vi "rsscope_core_global.vi"() -> ()   [LabVIEW 2018] (continued)
"Write Callback"="", "Supported Models"="", "Instrument Options"="K4", "Flags"=0, "Help"="Specifies a step to trigger on each n-th cycle inside the given range. This allows for specific triggering if slot multiplexing is used.\n\nAvailable Repeated Capabilities:\nTrigger: TrigA, TrigB, TrigR\r\n\nRemote-control command(s):\nTRIGger<m>:FLXRay:CSTep"}, {"Level"=3, "Class Only"=FALSE, "Identifier"="RSSCOPE_ATTR_PROTOCOL_FLEXRAY_TRIGGER_SYMBOL", "Descriptive Name"="Protocol FlexRay Trigger Symbol", "Data Type"=0, "Command"="TRIG{Trigger}:FLXR:SYMB", "Access"=2, "Range Table"="rsscope_rngFlexRaySymbol", "Read Callback"="", "Write Callback"="", "Supported Models"="", "Instrument Options"="K4", "Flags"=0, "Help"="Selects the trigger on symbol or on a wakeup pattern.\n\nAvailable Repeated Capabilities:\nTrigger: TrigA, TrigB, TrigR\r\n\nRemote-control command(s):\nTRIGger<m>:FLXRay:SYMBol"}, {"Level"=3, "Class Only"=TRUE, "Identifier"="", "Descriptive Name"="Indicator Bits", "Data Type"=0, "Command"="", "Access"=0, "Range Table"="", "Read Callback"="", "Write Callback"="", "Supported Models"="", "Instrument Options"="", "Flags"=0, "Help"="Configures indicator bits."}, {"Level"=4, "Class Only"=FALSE, "Identifier"="RSSCOPE_ATTR_PROTOCOL_FLEXRAY_TRIGGER_PAYLOAD_PREAMBLE", "Descriptive Name"="Protocol FlexRay Trigger Payload Preamble", "Data Type"=0, "Command"="TRIG{Trigger}:FLXR:PLPR", "Access"=2, "Range Table"="rsscope_rngFlexRayIndicatorBits", "Read Callback"="", "Write Callback"="", "Supported Models"="", "Instrument Options"="K4", "Flags"=0, "Help"="Triggers on the payload preamble indicator bit that indicates a Network Management Vector in the payload segment.\n\nAvailable Repeated Capabilities:\nTrigger: TrigA, TrigB, TrigR\r\n\nRemote-control command(s):\nTRIGger<m>:FLXRay:PLPReamble"}, {"Level"=4, "Class Only"=FALSE, "Identifier"="RSSCOPE_ATTR_PROTOCOL_FLEXRAY_TRIGGER_NULL_FRAME", "Descriptive Name"="Protocol FlexRay Trigger Null Frame", "Data Type"=0, "Command"="TRIG{Trigger}:FLXR:NUFR", "Access"=2, "Range Table"="rsscope_rngFlexRayIndicatorBits", "Read Callback"="", "Write Callback"="", "Supported Models"="", "Instrument Options"="K4", "Flags"=0, "Help"="Triggers on the null frame indicator bit, a frame without usable data.\n\nAvailable Repeated Capabilities:\nTrigger: TrigA, TrigB, TrigR\r\n\nRemote-control command(s):\nTRIGger<m>:FLXRay:NUFRame"}, {"Level"=4, "Class Only"=FALSE, "Identifier"="RSSCOPE_ATTR_PROTOCOL_FLEXRAY_TRIGGER_SYNC_FRAME", "Descriptive Name"="Protocol FlexRay Trigger Sync Frame", "Data Type"=0, "Command"="TRIG{Trigger}:FLXR:SYFR", "Access"=2, "Range Table"="rsscope_rngFlexRayIndicatorBits", "Read Callback"="", "Write Callback"="", "Supported Models"="", "Instrument Options"="K4", "Flags"=0, "Help"="Triggers on the sync frame used for synchronization of the FlexRay system. Only sync nodes can send this frame type.\n\nAvailable Repeated Capabilities:\nTrigger: TrigA, TrigB, TrigR\r\n\nRemote-control command(s):\nTRIGger<m>:FLXRay:SYFRame"}, {"Level"=4, "Class Only"=FALSE, "Identifier"="RSSCOPE_ATTR_PROTOCOL_FLEXRAY_TRIGGER_STARTUP_FRAME", "Descriptive Name"="Protocol FlexRay Trigger Startup Frame", "Data Type"=0, "Command"="TRIG{Trigger}:FLXR:STFR", "Access"=2, "Range Table"="rsscope_rngFlexRayIndicatorBits", "Read Callback"="", "Write Callback"="", "Supported Models"="", "Instrument Options"="K4", "Flags"=0, "Help"="Triggers on startup frames used for startup of the network. Only specific start nodes can send this frame type.\n\nAvailable Repeated Capabilities:\nTrigger: TrigA, TrigB, TrigR\r\n\nRemote-control command(s):\nTRIGger<m>:FLXRay:STFRame"}, {"Level"=3, "Class Only"=TRUE, "Identifier"="", "Descriptive Name"="Frame", "Data Type"=0, "Command"="", "Access"=0, "Range Table"="", "Read Callback"="", "Write Callback"="", "Supported Models"="", "Instrument Options"="", "Flags"=0, "Help"="Configures Flex Ray frame."}, {"Level"=4, "Class Only"=FALSE, "Identifier"="RSSCOPE_ATTR_PROTOCOL_FLEXRAY_TRIGGER_FRAME_CONDITION", "Descriptive Name"="Protocol FlexRay Trigger Frame Condition", "Data Type"=0, "Command"="TRIG{Trigger}:FLXR:FCON", "Access"=2, "Range Table"="rsscope_rngFlexRayCondition", "Read Callback"="", "Write Callback"="", "Supported Models"="", "Instrument Options"="K4", "Flags"=0, "Help"="Sets the operator to set a frame ID or a frame ID range.\n\nAvailable Repeated Capabilities:\nTrigger: TrigA, TrigB, TrigR\r\n\nRemote-control command(s):\nTRIGger<m>:FLXRay:FCONdition"}, {"Level"=4, "Class Only"=FALSE, "Identifier"="RSSCOPE_ATTR_PROTOCOL_FLEXRAY_TRIGGER_PATTERN_FRAME_MIN", "Descriptive Name"="Protocol FlexRay Trigger Pattern Frame Min", "Data Type"=2, "Command"="TRIG{Trigger}:FLXR:FMIN", "Access"=2, "Range Table"="", "Read Callback"="", "Write Callback"="", "Supported Models"="", "Instrument Options"="K4", "Flags"=0, "Help"="Specifies a frame identifier pattern - the number of the slot - or sets the start value of an identifier range.\n\nAvailable Repeated Capabilities:\nTrigger: TrigA, TrigB, TrigR\r\n\nRemote-control command(s):\nTRIGger<m>:FLXRay:FMIN"}, {"Level"=4, "Class Only"=FALSE, "Identifier"="RSSCOPE_ATTR_PROTOCOL_FLEXRAY_TRIGGER_PATTERN_FRAME_MAX", "Descriptive Name"="Protocol FlexRay Trigger Pattern Frame Max", "Data Type"=2, "Command"="TRIG{Trigger}:FLXR:FMAX", "Access"=2, "Range Table"="", "Read Callback"="", "Write Callback"="", "Supported Models"="", "Instrument Options"="K4", "Flags"=0, "Help"="Sets the end value of an identifier range.\n\nAvailable Repeated Capabilities:\nTrigger: TrigA, TrigB, TrigR\r\n\nRemote-control command(s):\nTRIGger<m>:FLXRay:FMAX"}, {"Level"=3, "Class Only"=TRUE, "Identifier"="", "Descriptive Name"="Data", "Data Type"=0, "Command"="", "Access"=0, "Range Table"="", "Read Callback"="", "Write Callback"="", "Supported Models"="", "Instrument Options"="", "Flags"=0, "Help"="Configures Flex ray data."}, {"Level"=4, "Class Only"=FALSE, "Identifier"="RSSCOPE_ATTR_PROTOCOL_FLEXRAY_TRIGGER_DATA_CONDITION", "Descriptive Name"="Protocol FlexRay Trigger Data Condition", "Data Type"=0, "Command"="TRIG{Trigger}:FLXR:DCON", "Access"=2, "Range Table"="rsscope_rngFlexRayCondition", "Read Callback"="", "Write Callback"="", "Supported Models"="", "Instrument Options"="K4", "Flags"=0, "Help"="Sets the operator to set a specific data pattern or a data pattern range.\n\nAvailable Repeated Capabilities:\nTrigger: TrigA, TrigB, TrigR\r\n\nRemote-control command(s):\nTRIGger<m>:FLXRay:DCONdition"}, {"Level"=4, "Class Only"=FALSE, "Identifier"="RSSCOPE_ATTR_PROTOCOL_FLEXRAY_TRIGGER_PATTERN_DATA_MIN", "Descriptive Name"="Protocol FlexRay Trigger Pattern Data Min", "Data Type"=2, "Command"="TRIG{Trigger}:FLXR:DMIN", "Access"=2, "Range Table"="", "Read Callback"="", "Write Callback"="", "Supported Models"="", "Instrument Options"="K4", "Flags"=0, "Help"="Specifies a data pattern, or sets the start value of a data pattern range.\n\nAvailable Repeated Capabilities:\nTrigger: TrigA, TrigB, TrigR\r\n\nRemote-control command(s):\nTRIGger<m>:FLXRay:DMIN"}, {"Level"=4, "Class Only"=FALSE, "Identifier"="RSSCOPE_ATTR_PROTOCOL_FLEXRAY_TRIGGER_PATTERN_DATA_MAX", "Descriptive Name"="Protocol FlexRay Trigger Pattern Data Max", "Data Type"=2, "Command"="TRIG{Trigger}:FLXR:DMAX", "Access"=2, "Range Table"="", "Read Callback"="", "Write Callback"="", "Supported Models"="", "Instrument Options"="K4", "Flags"=0, "Help"="Sets the end value of an data range.\n\nAvailable Repeated Capabilities:\nTrigger: TrigA, TrigB, TrigR\r\n\nRemote-control command(s):\nTRIGger<m>:FLXRay:DMAX"}, {"Level"=3, "Class Only"=TRUE, "Identifier"="", "Descriptive Name"="Payload Length", "Data Type"=0, "Command"="", "Access"=0, "Range Table"="", "Read Callback"="", "Write Callback"="", "Supported Models"="", "Instrument Options"="", "Flags"=0, "Help"="Configures Flex Ray Payload Length."}, {"Level"=4, "Class Only"=FALSE, "Identifier"="RSSCOPE_ATTR_PROTOCOL_FLEXRAY_TRIGGER_PAYLOAD_LENGTH_CONDITION", "Descriptive Name"="Protocol FlexRay Trigger Payload Length Condition", "Data Type"=0, "Command"="TRIG{Trigger}:FLXR:PCON", "Access"=2, "Range Table"="rsscope_rngFlexRayCondition", "Read Callback"="", "Write Callback"="", "Supported Models"="", "Instrument Options"="K4", "Flags"=0, "Help"="Sets the operator for the payload length trigger setting. You can defined an exact value, or a range.\n\nAvailable Repeated Capabilities:\nTrigger: TrigA, TrigB, TrigR\r\n\nRemote-control command(s):\nTRIGger<m>:FLXRay:PCONdition"}, {"Level"=4, "Class Only"=FALSE, "Identifier"="RSSCOPE_ATTR_PROTOCOL_FLEXRAY_TRIGGER_PAYLOAD_MIN", "Descriptive Name"="Protocol FlexRay Trigger Payload Min", "Data Type"=0, "Command"="TRIG{Trigger}:FLXR:PMIN", "Access"=2, "Range Table"="rsscope_rngFlexRayPayloadMinMax", "Read Callback"="", "Write Callback"="", "Supported Models"="", "Instrument Options"="K4", "Flags"=0, "Help"="Specifies a payload length - the number of words in the payload segment - or sets the start value of an payload length range. Information is transmitted in 2-byte words, so the number of data bytes in the payload segment is twice the payload length.\n\nAvailable Repeated Capabilities:\nTrigger: TrigA, TrigB, TrigR\r\n\nRemote-control command(s):\nTRIGger<m>:FLXRay:PMIN"}, {"Level"=4, "Class Only"=FALSE, "Identifier"="RSSCOPE_ATTR_PROTOCOL_FLEXRAY_TRIGGER_PAYLOAD_MAX", "Descriptive Name"="Protocol FlexRay Trigger Payload Max", "Data Type"=0, "Command"="TRIG{Trigger}:FLXR:PMAX", "Access"=2, "Range Table"="rsscope_rngFlexRayPayloadMinMax", "Read Callback"="", "Write Callback"="", "Supported Models"="", "Instrument Options"="K4", "Flags"=0, "Help"="Sets the end value of a payload length range.\n\nAvailable Repeated Capabilities:\nTrigger: TrigA, TrigB, TrigR\r\n\nRemote-control command(s):\nTRIGger<m>:FLXRay:PMAX"}, {"Level"=3, "Class Only"=TRUE, "Identifier"="", "Descriptive Name"="Cycle Count", "Data Type"=0, "Command"="", "Access"=0, "Range Table"="", "Read Callback"="", "Write Callback"="", "Supported Models"="", "Instrument Options"="", "Flags"=0, "Help"="Configures Flex Ray Cycle Count."}, {"Level"=4, "Class Only"=FALSE, "Identifier"="RSSCOPE_ATTR_PROTOCOL_FLEXRAY_TRIGGER_CYCLE_COUNT_CONDITION", "Descriptive Name"="Protocol FlexRay Trigger Cycle Count Condition", "Data Type"=0, "Command"="TRIG{Trigger}:FLXR:CEN", "Access"=2, "Range Table"="rsscope_rngFlexRayCondition", "Read Callback"="", "Write Callback"="", "Supported Models"="", "Instrument Options"="K4", "Flags"=0, "Help"="Sets the operator to define a cycle count or a cycle count range.\n\nAvailable Repeated Capabilities:\nTrigger: TrigA, TrigB, TrigR\r\n\nRemote-control command(s):\nTRIGger<m>:FLXRay:CENable"}, {"Level"=4, "Class Only"=FALSE, "Identifier"="RSSCOPE_ATTR_PROTOCOL_FLEXRAY_TRIGGER_CYCLE_MIN", "Descriptive Name"="Protocol FlexRay Trigger Cycle Min", "Data Type"=0, "Command"="TRIG{Trigger}:FLXR:CMIN", "Access"=2, "Range Table"="rsscope_rngFlexRayCycleMinMax", "Read Callback"="", "Write Callback"="", "Supported Models"="", "Instrument Options"="K4", "Flags"=0, "Help"="Specifies a cycle count - the number of the current FlexRay cycle - or sets the start value of an cycle count range.\n\nAvailable Repeated Capabilities:\nTrigger: TrigA, TrigB, TrigR\r\n\nRemote-control command(s):\nTRIGger<m>:FLXRay:CMIN"}, {"Level"=4, "Class Only"=FALSE, "Identifier"="RSSCOPE_ATTR_PROTOCOL_FLEXRAY_TRIGGER_CYCLE_MAX", "Descriptive Name"="Protocol FlexRay Trigger Cycle Max", "Data Type"=0, "Command"="TRIG{Trigger}:FLXR:CMAX", "Access"=2, "Range Table"="rsscope_rngFlexRayCycleMinMax", "Read Callback"="", "Write Callback"="", "Supported Models"="", "Instrument Options"="K4", "Flags"=0, "Help"="Sets the end value of a cycle count range.\n\nAvailable Repeated Capabilities:\nTrigger: TrigA, TrigB, TrigR\r\n\nRemote-control command(s):\nTRIGger<m>:FLXRay:CMAX"}, {"Level"=3, "Class Only"=TRUE, "Identifier"="", "Descriptive Name"="Data Position", "Data Type"=0, "Command"="", "Access"=0, "Range Table"="", "Read Callback"="", "Write Callback"="", "Supported Models"="", "Instrument Options"="", "Flags"=0, "Help"="Configures Flex Ray Data Position."}, {"Level"=4, "Class Only"=FALSE, "Identifier"="RSSCOPE_ATTR_PROTOCOL_FLEXRAY_TRIGGER_DATA_POSITION_CONDITION", "Descriptive Name"="Protocol FlexRay Trigger Data Position Condition", "Data Type"=0, "Command"="TRIG{Trigger}:FLXR:DPOP", "Access"=2, "Range Table"="rsscope_rngFlexRayCondition", "Read Callback"="", "Write Callback"="", "Supported Models"="", "Instrument Options"="K4", "Flags"=0, "Help"="Sets the operator for the data position. You can defined an exact position, or a position range.\n\nAvailable Repeated Capabilities:\nTrigger: TrigA, TrigB, TrigR\r\n\nRemote-control command(s):\nTRIGger<m>:FLXRay:DPOPerator"}, {"Level"=4, "Class Only"=FALSE, "Identifier"="RSSCOPE_ATTR_PROTOCOL_FLEXRAY_TRIGGER_DATA_POSITION_MIN", "Descriptive Name"="Protocol FlexRay Trigger Data Position Min", "Data Type"=0, "Command"="TRIG{Trigger}:FLXR:DPOS", "Access"=2, "Range Table"="rsscope_rngFlexRayPositionMinMax", "Read Callback"="", "Write Callback"="", "Supported Models"="", "Instrument Options"="K4", "Flags"=0, "Help"="Sets the number of data bytes to be skipped after start of the payload segment.\n\nAvailable Repeated Capabilities:\nTrigger: TrigA, TrigB, TrigR\r\n\nRemote-control command(s):\nTRIGger<m>:FLXRay:DPOSition"}, {"Level"=4, "Class Only"=FALSE, "Identifier"="RSSCOPE_ATTR_PROTOCOL_FLEXRAY_TRIGGER_DATA_POSITION_MAX", "Descriptive Name"="Protocol FlexRay Trigger Data Position Max", "Data Type"=0, "Command"="TRIG{Trigger}:FLXR:DPTO", "Access"=2, "Range Table"="rsscope_rngFlexRayPositionMinMax", "Read Callback"="", "Write Callback"="", "Supported Models"="", "Instrument Options"="K4", "Flags"=0, "Help"="Defines the last byte of interest.\n\nAvailable Repeated Capabilities:\nTrigger: TrigA, TrigB, TrigR\r\n\nRemote-control command(s):\nTRIGger<m>:FLXRay:DPTO"}, {"Level"=3, "Class Only"=TRUE, "Identifier"="", "Descriptive Name"="Error Conditions", "Data Type"=0, "Command"="", "Access"=0, "Range Table"="", "Read Callback"="", "Write Callback"="", "Supported Models"="", "Instrument Options"="", "Flags"=0, "Help"="Triggers on one or more errors in the frame."}, {"Level"=4, "Class Only"=FALSE, "Identifier"="RSSCOPE_ATTR_PROTOCOL_FLEXRAY_TRIGGER_FRAME_START_SEQUENCE_ERROR", "Descriptive Name"="Protocol FlexRay Trigger Frame Start Sequence Error", "Data Type"=3, "Command"="TRIG{Trigger}:FLXR:FSS", "Access"=2, "Range Table"="", "Read Callback"="", "Write Callback"="", "Supported Models"="", "Instrument Options"="K4", "Flags"=0, "Help"="Triggers on Error in a Frame Start Sequence. FSS follows the Transmission Start Sequence TSS at the beginning of each frame.\n\nAvailable Repeated Capabilities:\nTrigger: TrigA, TrigB, TrigR\r\n\nRemote-control command(s):\nTRIGger<m>:FLXRay:FSSerror"}, {"Level"=4, "Class Only"=FALSE, "Identifier"="RSSCOPE_ATTR_PROTOCOL_FLEXRAY_TRIGGER_BYTE_START_SEQUENCE_ERROR", "Descriptive Name"="Protocol FlexRay Trigger Byte Start Sequence Error", "Data Type"=3, "Command"="TRIG{Trigger}:FLXR:BSS", "Access"=2, "Range Table"="", "Read Callback"="", "Write Callback"="", "Supported Models"="", "Instrument Options"="K4", "Flags"=0, "Help"="Triggers on error in SyteStart Sequence. The BSS is transmitted before each byte.\n\nAvailable Repeated Capabilities:\nTrigger: TrigA, TrigB, TrigR\r\n\nRemote-control command(s):\nTRIGger<m>:FLXRay:BSSerror"}, {"Level"=4, "Class Only"=FALSE, "Identifier"="RSSCOPE_ATTR_PROTOCOL_FLEXRAY_TRIGGER_FRAME_END_SEQUENCE_ERROR", "Descriptive Name"="Protocol FlexRay Trigger Frame End Sequence Error", "Data Type"=3, "Command"="TRIG{Trigger}:FLXR:FES", "Access"=2, "Range Table"="", "Read Callback"="", "Write Callback"="", "Supported Models"="", "Instrument Options"="K4", "Flags"=0, "Help"="Triggers on error in Frame End Sequence. FES indicates the end of each frame.\n\nAvailable Repeated Capabilities:\nTrigger: TrigA, TrigB, TrigR\r\n\nRemote-control command(s):\nTRIGger<m>:FLXRay:FESerror"}, {"Level"=4, "Class Only"=FALSE, "Identifier"="RSSCOPE_ATTR_PROTOCOL_FLEXRAY_TRIGGER_HEADER_CRC_ERROR", "Descriptive Name"="Protocol FlexRay Trigger Header CRC Error", "Data Type"=3, "Command"="TRIG{Trigger}:FLXR:HCRC", "Access"=2, "Range Table"="", "Read Callback"="", "Write Callback"="", "Supported Models"="", "Instrument Options"="K4", "Flags"=0, "Help"="Triggers on error in the Cyclic Redundancy Check of the header data (mainly frame ID and payload length).\n\nAvailable Repeated Capabilities:\nTrigger: TrigA, TrigB, TrigR\r\n\nRemote-control command(s):\nTRIGger<m>:FLXRay:HCRCerror"}, {"Level"=4, "Class Only"=FALSE, "Identifier"="RSSCOPE_ATTR_PROTOCOL_FLEXRAY_TRIGGER_PAYLOAD_CRC_ERROR", "Descriptive Name"="Protocol FlexRay Trigger Payload CRC Error", "Data Type"=3, "Command"="TRIG{Trigger}:FLXR:PCRC", "Access"=2, "Range Table"="", "Read Callback"="", "Write Callback"="", "Supported Models"="", "Instrument Options"="K4", "Flags"=0, "Help"="Triggers on error in the Cyclic Redundancy Check of the payload data.\n\nAvailable Repeated Capabilities:\nTrigger: TrigA, TrigB, TrigR\r\n\nRemote-control command(s):\nTRIGger<m>:FLXRay:PCRCerror"}, {"Level"=2, "Class Only"=TRUE, "Identifier"="", "Descriptive Name"="Audio Signals", "Data Type"=0, "Command"="", "Access"=0, "Range Table"="", "Read Callback"="", "Write Callback"="", "Supported Models"="", "Instrument Options"="", "Flags"=0, "Help"="Configures Audio Signals trigger settings."}, {"Level"=3, "Class Only"=FALSE, "Identifier"="RSSCOPE_ATTR_PROTOCOL_AUDIO_TRIGGER_TYPE", "Descriptive Name"="Protocol Audio Trigger Type", "Data Type"=0, "Command"="TRIG:I2S:TYPE", "Access"=2, "Range Table"="rsscope_rngAudioTriggerType", "Read Callback"="", "Write Callback"="", "Supported Models"="", "Instrument Options"="", "Flags"=0, "Help"="This attribute select the trigger type.\n\nAvailable Repeated Capabilities:\nNone\n\nRemote-control command(s):\nTRIGger<m>:I2S:TYPE"}, {"Level"=3, "Class Only"=FALSE, "Identifier"="RSSCOPE_ATTR_PROTOCOL_AUDIO_TRIGGER_WINDOW_LENGTH", "Descriptive Name"="Protocol Audio Trigger Window Length", "Data Type"=0, "Command"="TRIG:I2S:SOW", "Access"=2, "Range Table"="rsscope_rngProtocolAudioWindowLength", "Read Callback"="", "Write Callback"="", "Supported Models"="", "Instrument Options"="", "Flags"=0, "Help"="Sets the number of words that is used as time limit for the &apos;Window&apos; trigger type.\n\nAvailable Repeated Capabilities:\nNone\n\nRemote-control command(s):\nTRIGger<m>:I2S:SOWords"}, {"Level"=3, "Class Only"=FALSE, "Identifier"="RSSCOPE_ATTR_PROTOCOL_AUDIO_TRIGGER_WORD_SELECT_SLOPE", "Descriptive Name"="Protocol Audio Trigger Word Select Slope", "Data Type"=0, "Command"="TRIG:I2S:WSSL", "Access"=2, "Range Table"="rsscope_rngPolarity", "Read Callback"="", "Write Callback"="", "Supported Models"="", "Instrument Options"="", "Flags"=0, "Help"="Sets the edge of the WS or FSYNC signal as trigger condition.\n\nAvailable Repeated Capabilities:\nNone\n\nRemote-control command(s):\nTRIGger<m>:I2S:WSSLope"}, {"Level"=3, "Class Only"=TRUE, "Identifier"="", "Descriptive Name"="Condition Number", "Data Type"=0, "Command"="", "Access"=0, "Range Table"="", "Read Callback"="", "Write Callback"="", "Supported Models"="", "Instrument Options"="", "Flags"=0, "Help"="Specifies the condition number."}, {"Level"=4, "Class Only"=FALSE, "Identifier"="RSSCOPE_ATTR_PROTOCOL_AUDIO_TRIGGER_CHANNEL", "Descriptive Name"="Protocol Audio Trigger Channel", "Data Type"=0, "Command"="TRIG:I2S:TCON{ConditionNumber}:CHAN", "Access"=2, "Range Table"="rsscope_rngAudioChannel", "Read Callback"="", "Write Callback"="", "Supported Models"="", "Instrument Options"="", "Flags"=0, "Help"="Selects the audio channel on which the instrument looks for the specified data condition.\n\nAvailable Repeated Capabilities:\nConditionNumber: Con1, Con2, Con3, Con4\r\n\nRemote-control command(s):\nTRIGger<m>:I2S:TCONdition<n>:CHANnel"}, {"Level"=4, "Class Only"=FALSE, "Identifier"="RSSCOPE_ATTR_PROTOCOL_AUDIO_TRIGGER_CONDITION", "Descriptive Name"="Protocol Audio Trigger Condition", "Data Type"=0, "Command"="TRIG:I2S:TCON{ConditionNumber}:COND", "Access"=2, "Range Table"="rsscope_rngProtocolTriggerCondition", "Read Callback"="", "Write Callback"="", "Supported Models"="", "Instrument Options"="", "Flags"=0, "Help"="Sets the operator to set a specific pattern or a pattern range.\n\nAvailable Repeated Capabilities:\nConditionNumber: Con1, Con2, Con3, Con4\r\n\nRemote-control command(s):\nTRIGger<m>:I2S:TCONdition<n>:CONDtion"}, {"Level"=4, "Class Only"=FALSE, "Identifier"="RSSCOPE_ATTR_PROTOCOL_AUDIO_TRIGGER_PATTERN_MIN", "Descriptive Name"="Protocol Audio Trigger Pattern Min", "Data Type"=2, "Command"="TRIG:I2S:TCON{ConditionNumber}:DMIN", "Access"=2, "Range Table"="", "Read Callback"="", "Write Callback"="", "Supported Models"="", "Instrument Options"="", "Flags"=0, "Help"="Min:\nSets a data pattern, or sets the start value of a data pattern range. Enter the pattern MSB first and with Big endian byte order. \n\nValid Values: \nBinary pattern string consisting 1; 0; or X (any bit). The maximum pattern length is 8 bytes.\n\nAvailable Repeated Capabilities:\nConditionNumber: Con1, Con2, Con3, Con4\r\n\nRemote-control command(s):\nTRIGger<m>:I2S:TCONdition<n>:DMIN"}, {"Level"=4, "Class Only"=FALSE, "Identifier"="RSSCOPE_ATTR_PROTOCOL_AUDIO_TRIGGER_PATTERN_MAX", "Descriptive Name"="Protocol Audio Trigger Pattern Max", "Data Type"=2, "Command"="TRIG:I2S:TCON{ConditionNumber}:DMAX", "Access"=2, "Range Table"="", "Read Callback"="", "Write Callback"="", "Supported Models"="", "Instrument Options"="", "Flags"=0, "Help"="Max:\nSets the end value of an data range.\n\nValid Values: \nBinary pattern string consisting 1; 0; or X (any bit). The maximum pattern length is 8 bytes.\n\nAvailable Repeated Capabilities:\nConditionNumber: Con1, Con2, Con3, Con4\r\n\nRemote-control command(s):\nTRIGger<m>:I2S:TCONdition<n>:DMAX"}, {"Level"=2, "Class Only"=TRUE, "Identifier"="", "Descriptive Name"="MIL1553", "Data Type"=0, "Command"="", "Access"=0, "Range Table"="", "Read Callback"="", "Write Callback"="", "Supported Models"="", "Instrument Options"="", "Flags"=0, "Help"="Configures MIL1553 trigger settings."}, {"Level"=3, "Class Only"=FALSE, "Identifier"="RSSCOPE_ATTR_PROTOCOL_MIL1553_TRIGGER_MODE", "Descriptive Name"="Protocol MIL1553 Trigger Mode", "Data Type"=0, "Command"="TRIG{Trigger}:MILS:TYPE", "Access"=2, "Range Table"="rsscope_rngProtocolMIL1553TriggerMode", "Read Callback"="", "Write Callback"="", "Supported Models"="RTO|RTP", "Instrument Options"="", "Flags"=0, "Help"="Sets the trigger type for MIL-1553 analysis.\n\nAvailable Repeated Capabilities:\nTrigger: TrigA, TrigB, TrigR\r\n\nRemote-control command(s):\nTRIGger<m>:MILStd:TYPE"}, {"Level"=3, "Class Only"=FALSE, "Identifier"="RSSCOPE_ATTR_PROTOCOL_MIL1553_SYNC_TYPE", "Descriptive Name"="Protocol MIL1553 Sync Type", "Data Type"=0, "Command"="TRIG{Trigger}:MILS:TPSP", "Access"=2, "Range Table"="rsscope_rngProtocolMIL1553SyncType", "Read Callback"="", "Write Callback"="", "Supported Models"="RTO|RTP", "Instrument Options"="", "Flags"=0, "Help"="Sets the sync impulse/ word type to be triggered on.\n\nAvailable Repeated Capabilities:\nTrigger: TrigA, TrigB, TrigR\r\n\nRemote-control command(s):\nTRIGger<m>:MILStd:TPSPecifier"}, {"Level"=3, "Class Only"=TRUE, "Identifier"="", "Descriptive Name"="Data", "Data Type"=0, "Command"="", "Access"=0, "Range Table"="", "Read Callback"="", "Write Callback"="", "Supported Models"="", "Instrument Options"="", "Flags"=0, "Help"="Configures MIL1553 trigger data settings."}, {"Level"=4, "Class Only"=TRUE, "Identifier"="", "Descriptive Name"="Pattern", "Data Type"=0, "Command"="", "Access"=0, "Range Table"="", "Read Callback"="", "Write Callback"="", "Supported Models"="", "Instrument Options"="", "Flags"=0, "Help"="Configures MIL1553 trigger data pattern settings."}, {"Level"=5, "Class Only"=FALSE, "Identifier"="RSSCOPE_ATTR_PROTOCOL_MIL1553_TRIGGER_DATA_PATTERN_CONDITION", "Descriptive Name"="Protocol MIL1553 Trigger Data Pattern Condition", "Data Type"=0, "Command"="TRIG{Trigger}:MILS:DATA:DCON", "Access"=2, "Range Table"="rsscope_rngProtocolMIL1553DataOperator", "Read Callback"="", "Write Callback"="", "Supported Models"="RTO|RTP", "Instrument Options"="", "Flags"=0, "Help"="Sets the operator to set a specific data pattern.\n\nAvailable Repeated Capabilities:\nTrigger: TrigA, TrigB, TrigR\r\n\nRemote-control command(s):\nTRIGger<m>:MILStd:DATA:DCONdition"}, {"Level"=5, "Class Only"=FALSE, "Identifier"="RSSCOPE_ATTR_PROTOCOL_MIL1553_TRIGGER_DATA_PATTERN_MIN", "Descriptive Name"="Protocol MIL1553 Trigger Data Pattern Min", "Data Type"=2, "Command"="TRIG{Trigger}:MILS:DATA:DMIN", "Access"=2, "Range Table"="", "Read Callback"="", "Write Callback"="", "Supported Models"="RTO|RTP", "Instrument Options"="", "Flags"=0, "Help"="Specifies a data pattern or sets the start value of a data pattern range.\n\nAvailable Repeated Capabilities:\nTrigger: TrigA, TrigB, TrigR\r\n\nRemote-control command(s):\nTRIGger<m>:MILStd:DATA:DMIN"}, {"Level"=5, "Class Only"=FALSE, "Identifier"="RSSCOPE_ATTR_PROTOCOL_MIL1553_TRIGGER_DATA_PATTERN_MAX", "Descriptive Name"="Protocol MIL1553 Trigger Data Pattern Max", "Data Type"=2, "Command"="TRIG{Trigger}:MILS:DATA:DMAX", "Access"=2, "Range Table"="", "Read Callback"="", "Write Callback"="", "Supported Models"="RTO|RTP", "Instrument Options"="", "Flags"=0, "Help"="Sets the end value of a data pattern range if &apos;Data Pattern Condition&apos; is set to InRange or OutOfRange.\n\nAvailable Repeated Capabilities:\nTrigger: TrigA, TrigB, TrigR\r\n\nRemote-control command(s):\nTRIGger<m>:MILStd:DATA:DMAX"}, {"Level"=4, "Class Only"=TRUE, "Identifier"="", "Descriptive Name"="Index", "Data Type"=0, "Command"="", "Access"=0, "Range Table"="", "Read Callback"="", "Write Callback"="", "Supported Models"="", "Instrument Options"="", "Flags"=0, "Help"="Configures MIL1553 trigger data index settings."}, {"Level"=5, "Class Only"=FALSE, "Identifier"="RSSCOPE_ATTR_PROTOCOL_MIL1553_TRIGGER_DATA_INDEX_CONDITION", "Descriptive Name"="Protocol MIL1553 Trigger Data Index Condition", "Data Type"=0, "Command"="TRIG{Trigger}:MILS:DATA:ICON", "Access"=2, "Range Table"="rsscope_rngProtocolIndexCondition", "Read Callback"="", "Write Callback"="", "Supported Models"="RTO|RTP", "Instrument Options"="", "Flags"=0, "Help"="Sets the operator to set a specific range within this series of the data words that is considered for the analysis.\n\nAvailable Repeated Capabilities:\nTrigger: TrigA, TrigB, TrigR\r\n\nRemote-control command(s):\nTRIGger<m>:MILStd:DATA:ICONdition"}, {"Level"=5, "Class Only"=FALSE, "Identifier"="RSSCOPE_ATTR_PROTOCOL_MIL1553_TRIGGER_DATA_INDEX_MIN", "Descriptive Name"="Protocol MIL1553 Trigger Data Index Min", "Data Type"=0, "Command"="TRIG{Trigger}:MILS:DATA:IMIN", "Access"=2, "Range Table"="rsscope_rngProtocolMIL1553TriggerDataIndexRange", "Read Callback"="", "Write Callback"="", "Supported Models"="RTO|RTP", "Instrument Options"="", "Flags"=0, "Help"="Specifies an index or sets the start value of a data word series index range.\n\nAvailable Repeated Capabilities:\nTrigger: TrigA, TrigB, TrigR\r\n\nRemote-control command(s):\nTRIGger<m>:MILStd:DATA:IMIN"}, {"Level"=5, "Class Only"=FALSE, "Identifier"="RSSCOPE_ATTR_PROTOCOL_MIL1553_TRIGGER_DATA_INDEX_MAX", "Descriptive Name"="Protocol MIL1553 Trigger Data Index Max", "Data Type"=0, "Command"="TRIG{Trigger}:MILS:DATA:IMAX", "Access"=2, "Range Table"="rsscope_rngProtocolMIL1553TriggerDataIndexRange", "Read Callback"="", "Write Callback"="", "Supported Models"="RTO|RTP", "Instrument Options"="", "Flags"=0, "Help"="Sets the end value of a data word series index range if &apos;Data Index Condition&apos; is set to InRange.\n\nAvailable Repeated Capabilities:\nTrigger: TrigA, TrigB, TrigR\r\n\nRemote-control command(s):\nTRIGger<m>:MILStd:DATA:IMAX"}, {"Level"=4, "Class Only"=TRUE, "Identifier"="", "Descriptive Name"="RTA Pattern", "Data Type"=0, "Command"="", "Access"=0, "Range Table"="", "Read Callback"="", "Write Callback"="", "Supported Models"="", "Instrument Options"="", "Flags"=0, "Help"="Configures MIL1553 trigger data RTA pattern settings."}, {"Level"=5, "Class Only"=FALSE, "Identifier"="RSSCOPE_ATTR_PROTOCOL_MIL1553_TRIGGER_RTA_DATA_PATTERN_CONDITION", "Descriptive Name"="Protocol MIL1553 Trigger RTA Data Pattern Condition", "Data Type"=0, "Command"="TRIG{Trigger}:MILS:DATA:RCON", "Access"=2, "Range Table"="rsscope_rngProtocolMIL1553DataOperator", "Read Callback"="", "Write Callback"="", "Supported Models"="RTO|RTP", "Instrument Options"="", "Flags"=0, "Help"="Sets the operator to set a specific remote terminal address.\n\nAvailable Repeated Capabilities:\nTrigger: TrigA, TrigB, TrigR\r\n\nRemote-control command(s):\nTRIGger<m>:MILStd:DATA:RCONdition"}, {"Level"=5, "Class Only"=FALSE, "Identifier"="RSSCOPE_ATTR_PROTOCOL_MIL1553_TRIGGER_RTA_DATA_PATTERN_MIN", "Descriptive Name"="Protocol MIL1553 Trigger RTA Data Pattern Min", "Data Type"=2, "Command"="TRIG{Trigger}:MILS:DATA:RMIN", "Access"=2, "Range Table"="", "Read Callback"="", "Write Callback"="", "Supported Models"="RTO|RTP", "Instrument Options"="", "Flags"=0, "Help"="Specifies a remote terminal address or sets the start value of a remote terminal address range.\n\nAvailable Repeated Capabilities:\nTrigger: TrigA, TrigB, TrigR\r\n\nRemote-control command(s):\nTRIGger<m>:MILStd:DATA:RMIN"}, {"Level"=5, "Class Only"=FALSE, "Identifier"="RSSCOPE_ATTR_PROTOCOL_MIL1553_TRIGGER_RTA_DATA_PATTERN_MAX", "Descriptive Name"="Protocol MIL1553 Trigger RTA Data Pattern Max", "Data Type"=2, "Command"="TRIG{Trigger}:MILS:DATA:RMAX", "Access"=2, "Range Table"="", "Read Callback"="", "Write Callback"="", "Supported Models"="RTO|RTP", "Instrument Options"="", "Flags"=0, "Help"="Sets the end value of a data range if &apos;Condition&apos; is set to InRange or OutOfRange.\n\nAvailable Repeated Capabilities:\nTrigger: TrigA, TrigB, TrigR\r\n\nRemote-control command(s):\nTRIGger<m>:MILStd:DATA:RMAX"}, {"Level"=3, "Class Only"=TRUE, "Identifier"="", "Descriptive Name"="Command Status", "Data Type"=0, "Command"="", "Access"=0, "Range Table"="", "Read Callback"="", "Write Callback"="", "Supported Models"="", "Instrument Options"="", "Flags"=0, "Help"="Configures MIL1553 trigger command status word settings."}, {"Level"=4, "Class Only"=TRUE, "Identifier"="", "Descriptive Name"="Remote Terminal Address", "Data Type"=0, "Command"="", "Access"=0, "Range Table"="", "Read Callback"="", "Write Callback"="", "Supported Models"="", "Instrument Options"="", "Flags"=0, "Help"="Configures MIL1553 trigger remote terminal address settings."}, {"Level"=5, "Class Only"=FALSE, "Identifier"="RSSCOPE_ATTR_PROTOCOL_MIL1553_TRIGGER_RTA_PATTERN_CONDITION", "Descriptive Name"="Protocol MIL1553 Trigger RTA Pattern Condition", "Data Type"=0, "Command"="TRIG{Trigger}:MILS:CDST:RCON", "Access"=2, "Range Table"="rsscope_rngProtocolMIL1553RTAOperator", "Read Callback"="", "Write Callback"="", "Supported Models"="RTO|RTP", "Instrument Options"="", "Flags"=0, "Help"="Sets the operator to set a specific remote terminal address.\n\nAvailable Repeated Capabilities:\nTrigger: TrigA, TrigB, TrigR\r\n\nRemote-control command(s):\nTRIGger<m>:MILStd:CDST:RCONdition"}, {"Level"=5, "Class Only"=FALSE, "Identifier"="RSSCOPE_ATTR_PROTOCOL_MIL1553_TRIGGER_RTA_PATTERN_MIN", "Descriptive Name"="Protocol MIL1553 Trigger RTA Pattern Min", "Data Type"=2, "Command"="TRIG{Trigger}:MILS:CDST:RMIN", "Access"=2, "Range Table"="", "Read Callback"="", "Write Callback"="", "Supported Models"="RTO|RTP", "Instrument Options"="", "Flags"=0, "Help"="Specifies a remote terminal address or sets the start value of a remote terminal address range.\n\nAvailable Repeated Capabilities:\nTrigger: TrigA, TrigB, TrigR\r\n\nRemote-control command(s):\nTRIGger<m>:MILStd:CDST:RMIN"}, {"Level"=5, "Class Only"=FALSE, "Identifier"="RSSCOPE_ATTR_PROTOCOL_MIL1553_TRIGGER_RTA_PATTERN_MAX", "Descriptive Name"="Protocol MIL1553 Trigger RTA Pattern Max", "Data Type"=2, "Command"="TRIG{Trigger}:MILS:CDST:RMAX", "Access"=2, "Range Table"="", "Read Callback"="", "Write Callback"="", "Supported Models"="RTO|RTP", "Instrument Options"="", "Flags"=0, "Help"="Sets the end value of a data range if &apos;RTA Condition&apos; is set to InRange or OutOfRange.\n\nAvailable Repeated Capabilities:\nTrigger: TrigA, TrigB, TrigR\r\n\nRemote-control command(s):\nTRIGger<m>:MILStd:CDST:RMAX"}, {"Level"=4, "Class Only"=TRUE, "Identifier"="", "Descriptive Name"="Info", "Data Type"=0, "Command"="", "Access"=0, "Range Table"="", "Read Callback"="", "Write Callback"="", "Supported Models"="", "Instrument Options"="", "Flags"=0, "Help"="Configures MIL1553 trigger 11-Bit Information settings."}, {"Level"=5, "Class Only"=FALSE, "Identifier"="RSSCOPE_ATTR_PROTOCOL_MIL1553_TRIGGER_INFO_PATTERN_CONDITION", "Descriptive Name"="Protocol MIL1553 Trigger Info Pattern Condition", "Data Type"=0, "Command"="TRIG{Trigger}:MILS:CDST:ICON", "Access"=2, "Range Table"="rsscope_rngProtocolMIL1553InfoOperator", "Read Callback"="", "Write Callback"="", "Supported Models"="RTO|RTP", "Instrument Options"="", "Flags"=0, "Help"="Sets the operator to set a specific info for the 9th to 19th bit of a command or status word.\n\nAvailable Repeated Capabilities:\nTrigger: TrigA, TrigB, TrigR\r\n\nRemote-control command(s):\nTRIGger<m>:MILStd:CDST:ICONdition"}, {"Level"=5, "Class Only"=FALSE, "Identifier"="RSSCOPE_ATTR_PROTOCOL_MIL1553_TRIGGER_INFO_PATTERN_MIN", "Descriptive Name"="Protocol MIL1553 Trigger Info Pattern Min", "Data Type"=2, "Command"="TRIG{Trigger}:MILS:CDST:IMIN", "Access"=2, "Range Table"="", "Read Callback"="", "Write Callback"="", "Supported Models"="RTO|RTP", "Instrument Options"="", "Flags"=0, "Help"="Specifies an info or sets the start value of an info range.\n\nAvailable Repeated Capabilities:\nTrigger: TrigA, TrigB, TrigR\r\n\nRemote-control command(s):\nTRIGger<m>:MILStd:CDST:IMIN"}, {"Level"=5, "Class Only"=FALSE, "Identifier"="RSSCOPE_ATTR_PROTOCOL_MIL1553_TRIGGER_INFO_PATTERN_MAX", "Descriptive Name"="Protocol MIL1553 Trigger Info Pattern Max", "Data Type"=2, "Command"="TRIG{Trigger}:MILS:CDST:IMAX", "Access"=2, "Range Table"="", "Read Callback"="", "Write Callback"="", "Supported Models"="RTO|RTP", "Instrument Options"="", "Flags"=0, "Help"="Sets the end value of the info range if &apos;Info Condition&apos; is set to InRange or OutOfRange.\n\nAvailable Repeated Capabilities:\nTrigger: TrigA, TrigB, TrigR\r\n\nRemote-control command(s):\nTRIGger<m>:MILStd:CDST:IMAX"}, {"Level"=3, "Class Only"=TRUE, "Identifier"="", "Descriptive Name"="Command", "Data Type"=0, "Command"="", "Access"=0, "Range Table"="", "Read Callback"="", "Write Callback"="", "Supported Models"="", "Instrument Options"="", "Flags"=0, "Help"="Configures MIL1553 trigger command word settings."}, {"Level"=4, "Class Only"=FALSE, "Identifier"="RSSCOPE_ATTR_PROTOCOL_MIL1553_TRIGGER_COMMAND_TRANSMIT_RECEIVE", "Descriptive Name"="Protocol MIL1553 Trigger Command Transmit Receive", "Data Type"=0, "Command"="TRIG{Trigger}:MILS:CMD:TR", "Access"=2, "Range Table"="rsscope_rngProtocolMIL1553TriggerCommandTransmitReceive", "Read Callback"="", "Write Callback"="", "Supported Models"="RTO|RTP", "Instrument Options"="", "Flags"=0, "Help"="Triggers on a transmission mode.\n\nAvailable Repeated Capabilities:\nTrigger: TrigA, TrigB, TrigR\r\n\nRemote-control command(s):\nTRIGger<m>:MILStd:CMD:TR"}, {"Level"=4, "Class Only"=TRUE, "Identifier"="", "Descriptive Name"="Subaddress", "Data Type"=0, "Command"="", "Access"=0, "Range Table"="", "Read Callback"="", "Write Callback"="", "Supported Models"="", "Instrument Options"="", "Flags"=0, "Help"="Configures MIL1553 trigger subaddress settings."}, {"Level"=5, "Class Only"=FALSE, "Identifier"="RSSCOPE_ATTR_PROTOCOL_MIL1553_TRIGGER_SUBADDRESS_PATTERN_CONDITION", "Descriptive Name"="Protocol MIL1553 Trigger Subaddress Pattern Condition", "Data Type"=0, "Command"="TRIG{Trigger}:MILS:CMD:SCON", "Access"=2, "Range Table"="rsscope_rngProtocolMIL1553SubaddressOperator", "Read Callback"="", "Write Callback"="", "Supported Models"="RTO|RTP", "Instrument Options"="", "Flags"=0, "Help"="Sets the operator to set a specific subaddress/mode pattern.\n\nAvailable Repeated Capabilities:\nTrigger: TrigA, TrigB, TrigR\r\n\nRemote-control command(s):\nTRIGger<m>:MILStd:CMD:SCONdition"}, {"Level"=5, "Class Only"=FALSE, "Identifier"="RSSCOPE_ATTR_PROTOCOL_MIL1553_TRIGGER_SUBADDRESS_PATTERN_MIN", "Descriptive Name"="Protocol MIL1553 Trigger Subaddress Pattern Min", "Data Type"=2, "Command"="TRIG{Trigger}:MILS:CMD:SMIN", "Access"=2, "Range Table"="", "Read Callback"="", "Write Callback"="", "Supported Models"="RTO|RTP", "Instrument Options"="", "Flags"=0, "Help"="Specifies a subaddress or sets the start value of a subaddress range.\n\nAvailable Repeated Capabilities:\nTrigger: TrigA, TrigB, TrigR\r\n\nRemote-control command(s):\nTRIGger<m>:MILStd:CMD:SMIN"}, {"Level"=5, "Class Only"=FALSE, "Identifier"="RSSCOPE_ATTR_PROTOCOL_MIL1553_TRIGGER_SUBADDRESS_PATTERN_MAX", "Descriptive Name"="Protocol MIL1553 Trigger Subaddress Pattern Max", "Data Type"=2, "Command"="TRIG{Trigger}:MILS:CMD:SMAX", "Access"=2, "Range Table"="", "Read Callback"="", "Write Callback"="", "Supported Models"="RTO|RTP", "Instrument Options"="", "Flags"=0, "Help"="Sets the end value of the info subaddress if &apos;Subaddress Condition&apos; is set to InRange or OutOfRange.\n\nAvailable Repeated Capabilities:\nTrigger: TrigA, TrigB, TrigR\r\n\nRemote-control command(s):\nTRIGger<m>:MILStd:CMD:SMAX"}, {"Level"=4, "Class Only"=TRUE, "Identifier"="", "Descriptive Name"="RTA Pattern", "Data Type"=0, "Command"="", "Access"=0, "Range Table"="", "Read Callback"="", "Write Callback"="", "Supported Models"="", "Instrument Options"="", "Flags"=0, "Help"="Configures MIL1553 trigger RTA Pattern settings."}, {"Level"=5, "Class Only"=FALSE, "Identifier"="RSSCOPE_ATTR_PROTOCOL_MIL1553_TRIGGER_COMMAND_RTA_PATTERN_CONDITION", "Descriptive Name"="Protocol MIL1553 Trigger Command RTA Pattern Condition", "Data Type"=0, "Command"="TRIG{Trigger}:MILS:CMD:RCON", "Access"=2, "Range Table"="rsscope_rngProtocolMIL1553SubaddressOperator", "Read Callback"="", "Write Callback"="", "Supported Models"="RTO|RTP", "Instrument Options"="", "Flags"=0, "Help"="Sets the operator to define a remote terminal address.\n\nAvailable Repeated Capabilities:\nTrigger: TrigA, TrigB, TrigR\r\n\nRemote-control command(s):\nTRIGger<m>:MILStd:CMD:RCONdition"}, {"Level"=5, "Class Only"=FALSE, "Identifier"="RSSCOPE_ATTR_PROTOCOL_MIL1553_TRIGGER_COMMAND_RTA_PATTERN_MIN", "Descriptive Name"="Protocol MIL1553 Trigger Command RTA Pattern Min", "Data Type"=2, "Command"="TRIG{Trigger}:MILS:CMD:RMIN", "Access"=2, "Range Table"="", "Read Callback"="", "Write Callback"="", "Supported Models"="RTO|RTP", "Instrument Options"="", "Flags"=0, "Help"="Specify a remote terminal address or set the start value of a remote terminal address range.\n\nAvailable Repeated Capabilities:\nTrigger: TrigA, TrigB, TrigR\r\n\nRemote-control command(s):\nTRIGger<m>:MILStd:CMD:RMIN"}, {"Level"=5, "Class Only"=FALSE, "Identifier"="RSSCOPE_ATTR_PROTOCOL_MIL1553_TRIGGER_COMMAND_RTA_PATTERN_MAX", "Descriptive Name"="Protocol MIL1553 Trigger Command RTA Pattern Max", "Data Type"=2, "Command"="TRIG{Trigger}:MILS:CMD:RMAX", "Access"=2, "Range Table"="", "Read Callback"="", "Write Callback"="", "Supported Models"="RTO|RTP", "Instrument Options"="", "Flags"=0, "Help"="Set the end value of a data range  if &apos;Condition&apos; is set to InRange or OutOfRange.\n\nAvailable Repeated Capabilities:\nTrigger: TrigA, TrigB, TrigR\r\n\nRemote-control command(s):\nTRIGger<m>:MILStd:CMD:RMAX"}, {"Level"=4, "Class Only"=TRUE, "Identifier"="", "Descriptive Name"="Word Count", "Data Type"=0, "Command"="", "Access"=0, "Range Table"="", "Read Callback"="", "Write Callback"="", "Supported Models"="", "Instrument Options"="", "Flags"=0, "Help"="Configures 
